vi "VI Tree - time__ogtk.vi"   [LabVIEW 2009]
panel:
  # "[OpenG VI Tags] ***Do Not Remove***"
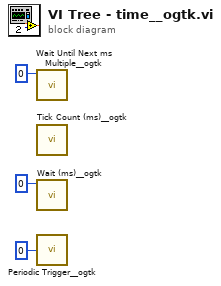
[diagram p0: block diagram]
diagram:
  n1 = call "Wait Until Next ms Multiple__ogtk.vi"("milliseconds to wait"=u32 0) -> ()  [unwired: 9 in, 2 out]
  n2 = call "Tick Count (ms)__ogtk.vi"() -> ()  [unwired: 10 in, 2 out]
  n3 = call "Wait (ms)__ogtk.vi"("milliseconds to wait"=u32 0) -> ()  [unwired: 9 in, 2 out]
  n4 = call "Periodic Trigger__ogtk.vi"("time (ms)"=u32 0) -> ()  [unwired: 12 in, 3 out]
